vi "G#Object_GetClassVersion.vi"(0 "reference in":refnum<class "G#Object.lvclass">, 5 "error in (no error)":errorcluster) -> (14 "reference out":refnum<class "G#Object.lvclass">, 16 "version":string, 19 "error out":errorcluster)   [LabVIEW 2017, in "G#Object.lvclass"]
doc: "Returns the version of the class specified by reference in."
uses:
  G#Object.lvclass
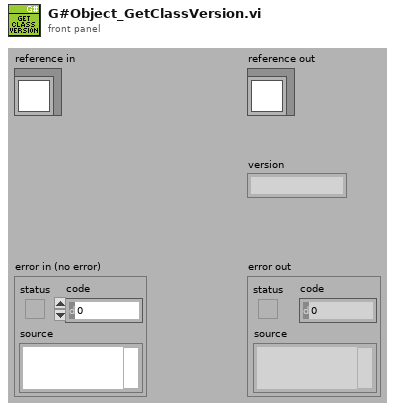
[diagram p1: front panel]
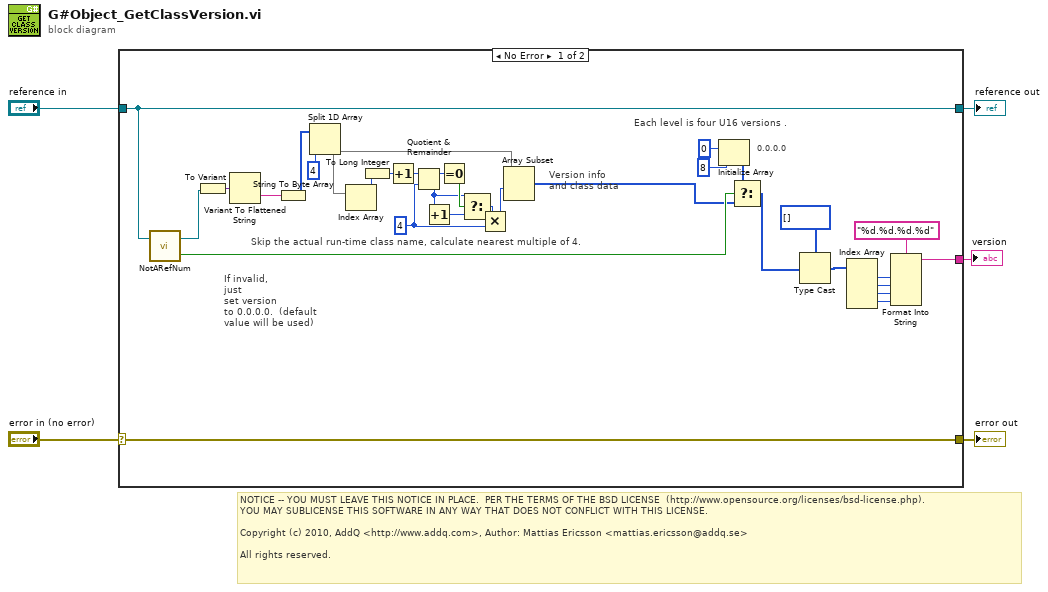
[diagram p0: block diagram]
diagram:
  # "NOTICE -- YOU MUST LEAVE THIS NOTICE IN PLACE.  PER THE TERMS OF THE BSD LICENSE  (http://www.opensource.org/licenses/bsd-license.php).\nYOU MAY SUBLICENSE THIS SOFTWARE IN ANY WAY THAT DOES NOT CONFLICT WITH THIS LICENSE.\n\nCopyright (c) 2010, AddQ <http://www.addq.com>, Author: Mattias Ericsson <mattias.ericsson@addq.se>\n\nAll rights reserved."
  n1 = case shown="No Error" "error in (no error)" {
    selector: "error in (no error)" -> [w17 w39]
    tunnel: [w17 w39] -> w4
    tunnel: [w19 w38] -> w2
    tunnel: "reference in" -> [w19 w38]
    tunnel: [w6 _] -> w1
    frame No Error {
      w27 = 4 ("y")
      # "0.0.0.0"
      # "If invalid,\njust\nset version\nto 0.0.0.0.  (default\nvalue will be used)"
      # "Each level is four U16 versions ."
      # "Version info\nand class data"
      # "Skip the actual run-time class name, calculate nearest multiple of 4."
      n2 = call-dynamic "NotARefNum.vi"("reference in"=w19) -> ("not a refnum?"=w18:bool, "reference out"=w20:refnum<class "G#Object.lvclass">)  [unwired: 1 in]
      n3 = To Variant(anything=w20) -> (Variant=w37:variant)
      n4 = Variant To Flattened String(Variant=w37) -> (data string=w26:string)  [unwired: 1 out]
      n5 = String To Byte Array(string=w26) -> (unsigned byte array=w30:u8[])
      n6 = Split 1D Array(array=w30, index=4 ("length")) -> (second subarray=w25:u8[])  [unwired: 1 out]
      n7 = Index Array(array=w25) -> (element=w36:u8)  [unwired: 1 in]
      n8 = To Long Integer(number=w36) -> (32bit integer=w24:i32)
      n9 = Increment(x=w24) -> (x+1=w23:i32)
      n10 = Quotient & Remainder(x=w23, y=w27) -> (x-y*floor(x/y)=w35:i32, floor(x/y)=w32:i32)
      n11 = Increment(x=w32) -> (x+1=w33:i32)
      n12 = Equal To 0?(x=w35) -> (x = 0?=w34:bool)
      n13 = Select(t=w32, s=w34, f=w33) -> (s? t:f=w29:i32)
      n14 = Multiply(x=w29, y=w27) -> (x*y=w28:i32)
      n15 = Array Subset(array=w25, index=w28) -> (w16:u8[])  [unwired: 1 in]
      n16 = Initialize Array(u8 0, 8 ("dimension size")) -> (w22:u8[])
      n17 = Select(t=w22, s=w18, f=w16) -> (s? t:f=w14:u8[])
      n18 = Type Cast(type=u16[] [], x=w14) -> (*(type *) &x=w12:u16[])
      n19 = Index Array(array=w12) -> (element #1=w11:u16, element #2=w10:u16, element #3=w9:u16, element #4=w8:u16)  [unwired: 4 in]
      n20 = Format Into String(format string="%d.%d.%d.%d", w11, w10, w9, w8) -> (resulting string=w6:string)  [unwired: 2 in, 1 out]
    }
    frame Error {
    }
  }
  "error out" <- w4
  "reference out" <- w2
  "version" <- w1
